vi "Sensor-Resistance-Sampling.vi"(1 "hold time (sec)":dbl=10.0 format="%#_13g", 2 "Gate step - extra milliseconds to wait":u32=20000, 3 "Current through sensor (A)":dbl format="%#_13g", 4 "Number of times measurement is done":i32=7, 6 "Number of heater steps":i32=7, 7 "Heater Step (V)":dbl=3.3) -> ()   [LabVIEW 2016]
uses:
  <vilib>/Utility/file.llb/Write To Spreadsheet File (DBL).vi
  <vilib>/Utility/file.llb/Read From Spreadsheet File (DBL).vi
  Driver/New driver/Agilent 415X Series.lvlib
panel:
  in  "number of samples per heater step":i32=10
  out "error out":errorcluster
  out "Voltage across heater (VSU 1 and SMU4)":dbl[][](graph)
  out "Voltage measured between SMU1 (Common) and SMU2":dbl[](graph)
  out "SPA VISA resource name":refnum<visa-resource-name>
  in  "1. SPA VISA resource name":refnum<visa-resource-name>="GPIB0::14::INSTR"
  in  "error in (no error)":errorcluster
  # "2. Heater Parameters"
  # "3. Repeat Entire Cycle"
  # "4. Timings \n(Should be same as those when sampling Thermopower)"
  # "5. Other measurement parameters"
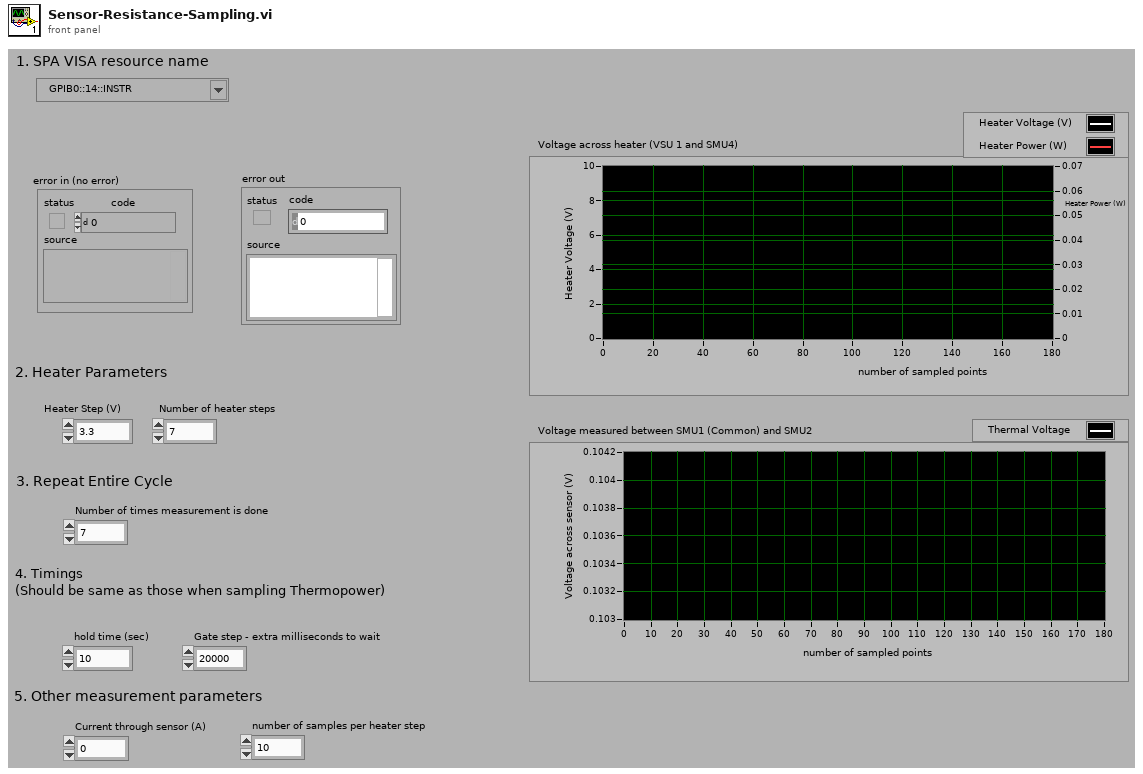
[diagram p1: front panel]
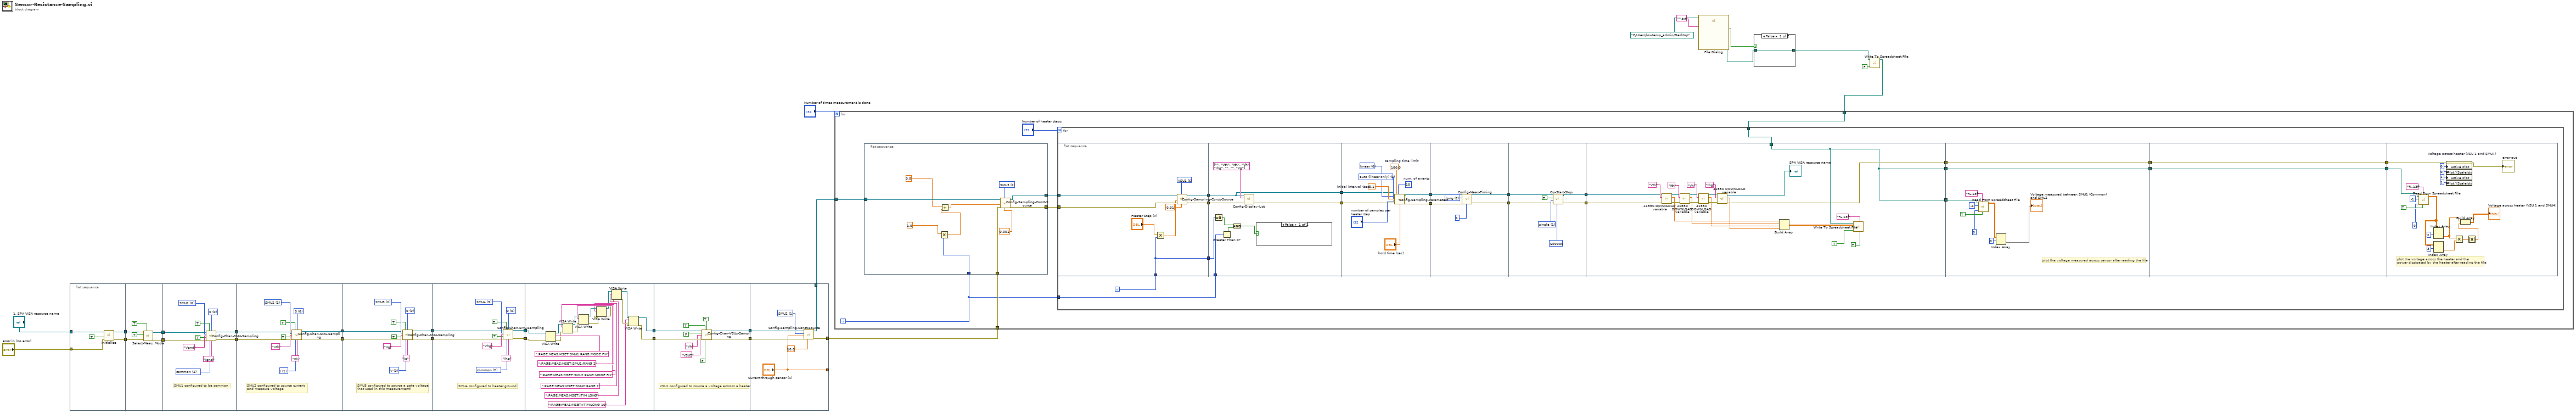
[diagram p0: block diagram]
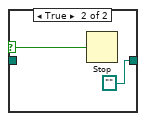
[diagram p2: hidden frame]
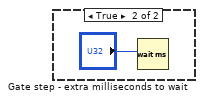
[diagram p3: hidden frame]
diagram:
  n1 = flat-sequence {
    tunnel: "error in (no error)" -> [w32]
    tunnel: "1. SPA VISA resource name" -> [w31]
    tunnel: [w30] -> w26
    tunnel: [w29] -> w25
    tunnel: w26 -> [w39]
    tunnel: w25 -> [w38]
    tunnel: [w35] -> w24
    tunnel: [w34] -> w23
    tunnel: w24 -> [w47]
    tunnel: w23 -> [w46]
    tunnel: [w45] -> w22
    tunnel: [w44] -> w21
    tunnel: w22 -> [w58]
    tunnel: w21 -> [w57]
    tunnel: [w56] -> w20
    tunnel: [w55] -> w19
    tunnel: w20 -> [w69]
    tunnel: w19 -> [w68]
    tunnel: [w67] -> w16
    tunnel: [w66] -> w15
    tunnel: w16 -> [w74]
    tunnel: [w75] -> w4
    tunnel: w15 -> [w73]
    tunnel: [w76] -> w2
    tunnel: w4 -> [w87]
    tunnel: [w84] -> w3
    tunnel: w2 -> [w86]
    tunnel: [w85] -> w1
    tunnel: w3 -> [w111]
    tunnel: w1 -> [w113]
    tunnel: [w112] -> w18
    tunnel: [w110] -> w17
    tunnel: w18 -> [w117]
    tunnel: w17 -> [w118]
    tunnel: [w116] -> w13
    tunnel: [w115] -> w12
    tunnel: ["Current through sensor (A)"] -> _
    frame #0 {
      n2 = call "Initialize.vi"("error in (no error)"=w32, "reset"=TRUE, "VISA resource name"=w31) -> ("error out"=w29:errorcluster, "VISA resource name out"=w30:refnum<visa-resource-name>)  [unwired: 2 in, 5 out]
    }
    frame #1 {
      n3 = call "Select-Meas. Mode.vi"("clear all channels"=TRUE, "error in (no error)"=w38, "measurement mode"=TRUE, "VISA resource name"=w39) -> ("error out"=w34:errorcluster, "VISA resource name out"=w35:refnum<visa-resource-name>)  [unwired: 1 in, 5 out]
    }
    frame #2 {
      w42 = 0 items=["0  ", "10K Ohms  ", "100K Ohms  ", "1M Ohms  "] ("series resistance *")
      w43 = 2 items=["V  ", "I  ", "  common  "] ("mode")
      w48 = 0 items=["SMU1  ", "SMU2  ", "SMU3  ", "SMU4  ", "SMU5  ", "SMU6  "] ("unit to configure")
      # "SMU1 configured to be common"
      n4 = call "Config-Chan-SMU-Sampling.vi"("VISA resource name in"=w47, "function"=TRUE, "series resistance *"=w42, "unit to configure"=w48, "V name (max 6 chars)"="Vgnd", "standby"=TRUE, "error in (no error)"=w46, "mode"=w43, "I name (max 6 chars)"="Ignd") -> ("VISA resource name out"=w45:refnum<visa-resource-name>, "error out"=w44:errorcluster)  [unwired: 5 out]
    }
    frame #3 {
      w52 = 0 items=["0  ", "10K Ohms  ", "100K Ohms  ", "1M Ohms  "] ("series resistance *")
      w54 = 1 items=["V  ", "I  ", "  common  "] ("mode")
      w59 = 1 items=["SMU1  ", "SMU2  ", "SMU3  ", "SMU4  ", "SMU5  ", "SMU6  "] ("unit to configure")
      # "SMU2 configured to source current \nand measure voltage"
      n5 = call "Config-Chan-SMU-Sampling.vi"("VISA resource name in"=w58, "function"=TRUE, "series resistance *"=w52, "unit to configure"=w59, "V name (max 6 chars)"="Vth", "standby"=TRUE, "error in (no error)"=w57, "mode"=w54, "I name (max 6 chars)"="Ith") -> ("VISA resource name out"=w56:refnum<visa-resource-name>, "error out"=w55:errorcluster)  [unwired: 5 out]
    }
    frame #4 {
      w63 = 0 items=["0  ", "10K Ohms  ", "100K Ohms  ", "1M Ohms  "] ("series resistance *")
      w65 = 0 items=["V  ", "I  ", "  common  "] ("mode")
      w70 = 2 items=["SMU1  ", "SMU2  ", "SMU3  ", "SMU4  ", "SMU5  ", "SMU6  "] ("unit to configure")
      # "SMU3 configured to source a gate voltage\n(not used in this measurement)"
      n6 = call "Config-Chan-SMU-Sampling.vi"("VISA resource name in"=w69, "function"=TRUE, "series resistance *"=w63, "unit to configure"=w70, "V name (max 6 chars)"="Vg", "standby"=TRUE, "error in (no error)"=w68, "mode"=w65, "I name (max 6 chars)"="Ig") -> ("VISA resource name out"=w67:refnum<visa-resource-name>, "error out"=w66:errorcluster)  [unwired: 5 out]
    }
    frame #5 {
      w78 = 0 items=["0  ", "10K Ohms  ", "100K Ohms  ", "1M Ohms  "] ("series resistance *")
      w80 = 2 items=["V  ", "I  ", "  common  "] ("mode")
      w81 = 3 items=["SMU1  ", "SMU2  ", "SMU3  ", "SMU4  ", "SMU5  ", "SMU6  "] ("unit to configure")
      # "SMU4 configured to heater ground"
      n7 = call "Config-Chan-SMU-Sampling.vi"("VISA resource name in"=w74, "function"=TRUE, "series resistance *"=w78, "unit to configure"=w81, "V name (max 6 chars)"="Vhg", "standby"=TRUE, "error in (no error)"=w73, "mode"=w80, "I name (max 6 chars)"="Ihg") -> ("VISA resource name out"=w75:refnum<visa-resource-name>, "error out"=w76:errorcluster)  [unwired: 5 out]
    }
    frame #6 {
      n8 = VISA Write(VISA resource name=w87, write buffer=":PAGE:MEAS:MSET:SMU1:RANG:MODE FIX", error in (no error)=w86) -> (VISA resource name out=w102:refnum<visa-resource-name>, error out=w99:errorcluster)  [unwired: 1 out]
      n9 = VISA Write(VISA resource name=w102, write buffer=":PAGE:MEAS:MSET:SMU1:RANG 2", error in (no error)=w99) -> (VISA resource name out=w101:refnum<visa-resource-name>, error out=w98:errorcluster)  [unwired: 1 out]
      n10 = VISA Write(VISA resource name=w101, write buffer=":PAGE:MEAS:MSET:SMU2:RANG:MODE FIX", error in (no error)=w98) -> (VISA resource name out=w100:refnum<visa-resource-name>, error out=w97:errorcluster)  [unwired: 1 out]
      n11 = VISA Write(VISA resource name=w100, write buffer=":PAGE:MEAS:MSET:SMU2:RANG 2", error in (no error)=w97) -> (VISA resource name out=w92:refnum<visa-resource-name>, error out=w91:errorcluster)  [unwired: 1 out]
      n12 = VISA Write(VISA resource name=w92, write buffer=":PAGE:MEAS:MSET:ITIM LONG", error in (no error)=w91) -> (VISA resource name out=w90:refnum<visa-resource-name>, error out=w89:errorcluster)  [unwired: 1 out]
      n13 = VISA Write(VISA resource name=w90, write buffer=":PAGE:MEAS:MSET:ITIM:LONG 10", error in (no error)=w89) -> (VISA resource name out=w84:refnum<visa-resource-name>, error out=w85:errorcluster)  [unwired: 1 out]
    }
    frame #7 {
      # "VSU1 configured to source a voltage accross a heater"
      n14 = call "Config-Chan-VSUs-Sampling.vi"("VISA session"=w111, "VSU1 function"=TRUE, "VSU2 standby"=TRUE, "VSU1 standby"=FALSE, "VSU1 V name \n(max 6 chars)"="Vh" ("V name (max 6 chars)"), "VSU2 V name \n(max 6 chars)"="VSU2" ("V name (max 6 chars)"), "error in (no error)"=w113, "VSU2 function"=FALSE) -> ("VISA resource name out"=w110:refnum<visa-resource-name>, "error out"=w112:errorcluster)  [unwired: 6 out]
    }
    frame #8 {
      w119 = u16 1 items=["SMU 1", "SMU2", "SMU3", "SMU4", "SMU5", "SMU6", "VSU1", "VSU2"] ("unit (SMU1:0)")
      n15 = call "Config-Sampling-Const-Source.vi"("compliance (SMUs only)"=10.0, "error in (no error)"=w117, "source (V or A)"="Current through sensor (A)", "unit (SMU1:0)"=w119, "VISA session"=w118) -> ("error out"=w115:errorcluster, "VISA resource name out"=w116:refnum<visa-resource-name>)  [unwired: 5 out]
    }
  }
  n16 = call "File Dialog"("start path"=path "C:/Users/lowtemp_admin/Desktop", "pattern (all files)"="*.txt") -> ("selected path"=w10:path, "cancelled"=w9:bool)  [unwired: 10 in, 2 out]
  n17 = case shown="False" w9 {
    selector: w9 -> [_ w123]
    tunnel: w10 -> [w121 _]
    tunnel: [w121 path ""] -> w6
    frame False {
    }
    frame True {
      n18 = Stop(stop? (T)=w123) -> ()
    }
  }
  n19 = call-poly <vilib>:"Write To Spreadsheet File.vi"("append to file? (new file:F)"=FALSE, "file path (dialog if empty)"=w6) -> ("new file path (Not A Path if cancelled)"=w5:path)  [unwired: 6 in]
  n20 = for {
    N: "Number of times measurement is done" -> [_]
    tunnel: w13 -> [w127]
    tunnel: w12 -> [w126]
    tunnel: w5 -> [w124]
    i -> [w125]
    n21 = flat-sequence {
      tunnel: w125 -> [w255]
      tunnel: [w260] -> w129
      tunnel: [w259] -> w128
      tunnel: w127 -> [w258]
      tunnel: w126 -> [w257]
      frame #0 {
        w261 = u16 2 items=["SMU 1", "SMU2", "SMU3", "SMU4", "SMU5", "SMU6", "VSU1", "VSU2"] ("unit (SMU1:0)")
        n22 = Multiply(x=1.0 ("Gate Start"), y=w255) -> (x*y=w254:dbl)
        n23 = Add(x=0.0 ("Gate Start"), y=w254) -> (x+y=w253:dbl)
        n24 = call "Config-Sampling-Const-Source.vi"("compliance (SMUs only)"=0.001, "error in (no error)"=w257, "source (V or A)"=w253, "unit (SMU1:0)"=w261, "VISA session"=w258) -> ("error out"=w259:errorcluster, "VISA resource name out"=w260:refnum<visa-resource-name>)  [unwired: 5 out]
      }
    }
    n25 = for {
      N: "Number of heater steps" -> [_]
      tunnel: w129 -> [w142]
      tunnel: w128 -> [w141]
      tunnel: w124 -> [w140]
      tunnel: w125 -> [w133]
      i -> [w143]
      n26 = flat-sequence {
        tunnel: [w161] -> w153
        tunnel: [w160] -> w152
        tunnel: w143 -> [w155]
        tunnel: w142 -> [w159]
        tunnel: w141 -> [w158]
        tunnel: [w155] -> w134
        tunnel: w153 -> [w170]
        tunnel: w152 -> [w168]
        tunnel: [w169] -> w151
        tunnel: [w168] -> w150
        tunnel: w134 -> [w164]
        tunnel: w133 -> [w163]
        tunnel: w151 -> [w176]
        tunnel: w150 -> [w175]
        tunnel: [w174] -> w149
        tunnel: [w173] -> w148
        tunnel: w149 -> [w187]
        tunnel: w148 -> [w186]
        tunnel: [w185] -> w147
        tunnel: [w184] -> w146
        tunnel: w147 -> [w193]
        tunnel: w146 -> [w192]
        tunnel: [w191] -> w145
        tunnel: [w190] -> w144
        tunnel: w145 -> [w200]
        tunnel: w144 -> [w199]
        tunnel: w140 -> [w201]
        tunnel: [w201] -> w139
        tunnel: [w201] -> w138
        tunnel: [w197] -> w136
        tunnel: w139 -> [w226]
        tunnel: [w224] -> w132
        tunnel: w138 -> [w224]
        tunnel: w136 -> [w221]
        tunnel: [w221] -> w131
        tunnel: [w231] -> w137
        tunnel: [w230] -> w135
        tunnel: w131 -> [w230]
        tunnel: w132 -> [w231]
        tunnel: w137 -> [w232]
        tunnel: w135 -> [w237]
        frame #0 {
          w162 = u16 6 items=["SMU 1", "SMU2", "SMU3", "SMU4", "SMU5", "SMU6", "VSU1", "VSU2"] ("unit (SMU1:0)")
          n27 = Multiply(x="Heater Step (V)", y=w155) -> (x*y=w156:dbl)
          n28 = call "Config-Sampling-Const-Source.vi"("compliance (SMUs only)"=0.01, "error in (no error)"=w158, "source (V or A)"=w156, "unit (SMU1:0)"=w162, "VISA session"=w159) -> ("error out"=w161:errorcluster, "VISA resource name out"=w160:refnum<visa-resource-name>)  [unwired: 5 out]
        }
        frame #1 {
          n29 = Equal To 0?(x=w164) -> (x = 0?=w165:bool)
          n30 = Greater Than 0?(x=w163) -> (x > 0?=w166:bool)
          n31 = And(x=w165, y=w166) -> (x .and. y?=w167:bool)
          n32 = call "Config-Display-List.vi"("error in (no error)"=w170, "list (max 8 elements)"=string[] ["", "Vth", "Ith", "Vh", "Ihg", "", "", "Vg"], "VISA session"=w168) -> ("error out"=w169:errorcluster)  [unwired: 1 in, 7 out]
          n33 = case shown="False" w167 {
            frame False {
            }
            frame True {
              n34 = Wait (ms)(milliseconds to wait="Gate step - extra milliseconds to wait") -> ()  [unwired: 1 out]
            }
          }
        }
        frame #2 {
          w177 = 100.0  # sampling time limit
          w178 = 0 items=["linear", "log 10", "log 25", "log 50", "thinned out"] ("mode (linear: 0)")
          w179 = 0 items=["auto (linear only)", "no limit", "set limit "] ("sampling time\n(linear/thinned-out only)")
          w180 = 0.1  # initial interval (sec)
          w181 = 10  # num. of events
          n35 = call "Config-Sampling-Parameters.vi"("VISA session"=w175, "mode (linear: 0)"=w178, "initial interval (sec)"=w180, "sampling time\n(linear/thinned-out only)"=w179, "number of samples"="number of samples per heater step", "error in (no error)"=w176, "sampling time limit"=w177, "num. of events"=w181, "hold time (sec)"="hold time (sec)") -> ("VISA resource name out"=w173:refnum<visa-resource-name>, "error out"=w174:errorcluster)  [unwired: 7 in, 10 out]
        }
        frame #3 {
          w189 = 2 items=["short  ", "medium  ", "long  "] ("integration time")
          n36 = call "Config-Meas-Timing.vi"("# PLCs for long integration time"=1, "error in (no error)"=w187, "integration time"=w189, "VISA session"=w186) -> ("error out"=w185:errorcluster, "VISA resource name out"=w184:refnum<visa-resource-name>)  [unwired: 2 in, 4 out]
        }
        frame #4 {
          w195 = 1 items=["stop  ", "single  ", "single-append  ", "stress start  ", "continuous  ", "standby on  ", "standby off  ", "zero  "] ("function (stop:0)")
          n37 = call "Op-Start-Stop.vi"("time to wait (30000ms)"=600000, "error in (no error)"=w193, "function (stop:0)"=w195, "wait until finish"=TRUE, "VISA resource name"=w192) -> ("error out"=w191:errorcluster, "VISA resource name out"=w190:refnum<visa-resource-name>)  [unwired: 5 out]
        }
        frame #5 {
          n38 = call "4155C DOWNLOAD variable.vi"("error in (no error)"=w200, "Variable name"="Vth", "VISA resource name in"=w199) -> ("error out"=w210:errorcluster, "Output data"=w203:dbl[], "VISA Resource Name out"=w213:refnum<visa-resource-name>)  [unwired: 2 out]
          n39 = call "4155C DOWNLOAD variable.vi"("error in (no error)"=w210, "Variable name"="Ith", "VISA resource name in"=w213) -> ("error out"=w209:errorcluster, "Output data"=w207:dbl[], "VISA Resource Name out"=w212:refnum<visa-resource-name>)  [unwired: 2 out]
          n40 = call "4155C DOWNLOAD variable.vi"("error in (no error)"=w209, "Variable name"="Vh", "VISA resource name in"=w212) -> ("error out"=w208:errorcluster, "Output data"=w206:dbl[], "VISA Resource Name out"=w211:refnum<visa-resource-name>)  [unwired: 2 out]
          n41 = call "4155C DOWNLOAD variable.vi"("error in (no error)"=w208, "Variable name"="Ihg", "VISA resource name in"=w211) -> ("error out"=w197:errorcluster, "Output data"=w205:dbl[], "VISA Resource Name out"=→"SPA VISA resource name":refnum<visa-resource-name>)  [unwired: 2 out]
          n42 = Build Array(w203, w207, w206, w205) -> (w204:dbl[][])
          n43 = call-poly <vilib>:"Write To Spreadsheet File.vi"("transpose? (no:F)"=TRUE, "format (%.3f)"="%.13f", "append to file? (new file:F)"=TRUE, "2D data"=w204, "file path (dialog if empty)"=w201) -> ()  [unwired: 1 in, 3 out]
        }
        frame #6 {
          # "plot the voltage measured across sensor after reading the file"
          n44 = call-poly <vilib>:"Read From Spreadsheet File.vi"("transpose (no:F)"=TRUE, "format (%.3f)"="%.13f", "max characters/row  (no limit:0)"=0, "number of rows (all:-1)"=-1, "file path (dialog if empty)"=w226) -> ("all rows"=w223:dbl[][])  [unwired: 6 out]
          n45 = Index Array(array=w223, index (row)=0) -> (element=→"Voltage measured between SMU1 (Common) and SMU2":dbl[])  [unwired: 1 in]
        }
        frame #7 {
        }
        frame #8 {
          # "plot the voltage across the heater and the \npower dissipated by the heater after reading the file"
          n46 = call-poly <vilib>:"Read From Spreadsheet File.vi"("transpose (no:F)"=TRUE, "format (%.3f)"="%.13f", "max characters/row  (no limit:0)"=0, "number of rows (all:-1)"=-1, "file path (dialog if empty)"=w232) -> ("all rows"=w245:dbl[][])  [unwired: 6 out]
          n47 = Index Array(array=w245, index (row)=2) -> (element=w239:dbl[])  [unwired: 1 in]
          n48 = Index Array(array=w245, index (row)=3) -> (element=w243:dbl[])  [unwired: 1 in]
          n49 = property on="Voltage across heater (VSU 1 and SMU4)" class="WFGraph (strict)"(error in=w237, "Active Plot"=u32 0, "Plot.YScaleIdx"=u32 0 ("Plot.Y Scale Index"), "Active Plot"=u32 1, "Plot.YScaleIdx"=u32 1 ("Plot.Y Scale Index")) -> (error out=→"error out":errorcluster)  [unwired: 1 in, 1 out]
          n50 = Multiply(x=w239, y=w243) -> (x*y=w242:dbl[])
          n51 = Absolute Value(x=w242) -> (abs(x)=w241:dbl[])
          n52 = Build Array(w239, w241) -> (→"Voltage across heater (VSU 1 and SMU4)":dbl[][])
        }
      }
    }
  }
